vi "MongoDB.DocumentFindAll.vi"(8 "error in (no error)":errorcluster, 11 "MongoDB.Collection in":refnum<class "MongoDB.Collection.lvclass">) -> (0 "error out":errorcluster, 2 "Results":string[](array[string]), 3 "MongoDB.Collection out":refnum<class "MongoDB.Collection.lvclass">)   [LabVIEW 2014, in "MongoDB.Collection.lvclass"]
uses:
  MongoDB.Collection.lvclass
  MongoDB.Collection.lvclass/MongoDB.Collection.ctl
  C:/Users/Richard/Documents/GitHub/mongo-labview-driver/CSharp/bin/MongoDB.Driver.Legacy.dll
  CSharp/bin/MongoDB.Driver.Legacy.dll
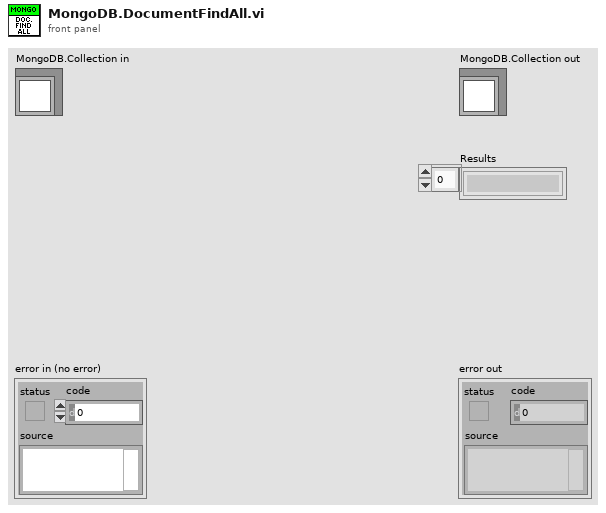
[diagram p1: front panel]
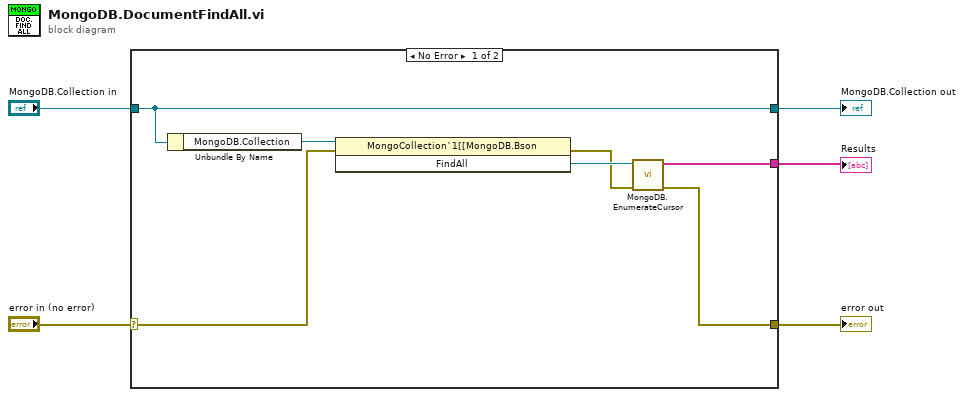
[diagram p0: block diagram]
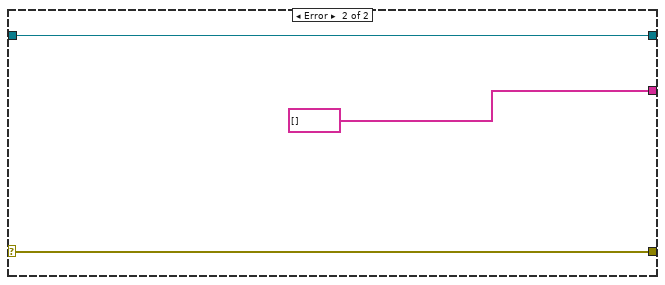
[diagram p2: hidden frame]
diagram:
  n1 = case shown="No Error" "error in (no error)" {
    selector: "error in (no error)" -> [w6 w15]
    tunnel: [w7 w15] -> w4
    tunnel: [w12 w14] -> w2
    tunnel: "MongoDB.Collection in" -> [w12 w14]
    tunnel: [w9 string[] [] ("Array")] -> w1
    frame No Error {
      n2 = Unbundle By Name(w12) -> ("MongoDB.Collection"=w11:refnum<k24>)
      n3 = invoke class="MongoCollection`1[[MongoDB.Bson" method="FindAll"(reference=w11, error in=w6) -> (error out=w8:errorcluster, "FindAll"=w10:refnum<k24>)  [unwired: 1 in, 1 out]
      n4 = call "MongoDB.EnumerateCursor.vi"("error in (no error)"=w8, "MongoDB.Cursor"=w10) -> ("error out"=w7:errorcluster, "Array"=w9:string[])  [unwired: 8 in]
    }
    frame Error {
    }
  }
  "error out" <- w4
  "MongoDB.Collection out" <- w2
  "Results" <- w1
